vi "gui-camera-status-converter.vi"(1 "xenics-status-cluster":T1, 2 "andor-status-cluster":T4={"Newton Init"=FALSE, "Newton Cooling"=FALSE, "Newton Parameters "=FALSE, "iDus Init"=FALSE, "iDus Cooling"=FALSE, "iDus Parameters"=FALSE, "Clara Init"=FALSE, "Clara Cooling"=FALSE, "Clara Parameters"=FALSE, "Newton Cooler StatusCode"=enum."N/A (0)", "iDus Cooler StatusCode"=enum."N/A (0)", "Clara Cooler StatusCode"=enum."DRV_TEMPERATURE_NOT_REACHED"}) -> (0 "general-camera-status":T2)   [LabVIEW 2017]
uses:
  <userlib>/atmcd32d.llb/Error Code Enum typedef.ctl
panel:
  # "Init"
  # "Cooling"
  # "Parameters"
  # "Xeva"
  # "Init"
  # "Cooling"
  # "Parameters"
  # "Newton"
  # "iDus"
  # "Clara"
  # "Xeva"
  # "Init"
  # "Cooling"
  # "Parameters"
  # "Newton"
  # "iDus"
  # "Clara"
  # "Clara"
  # "iDus"
  # "Newton"
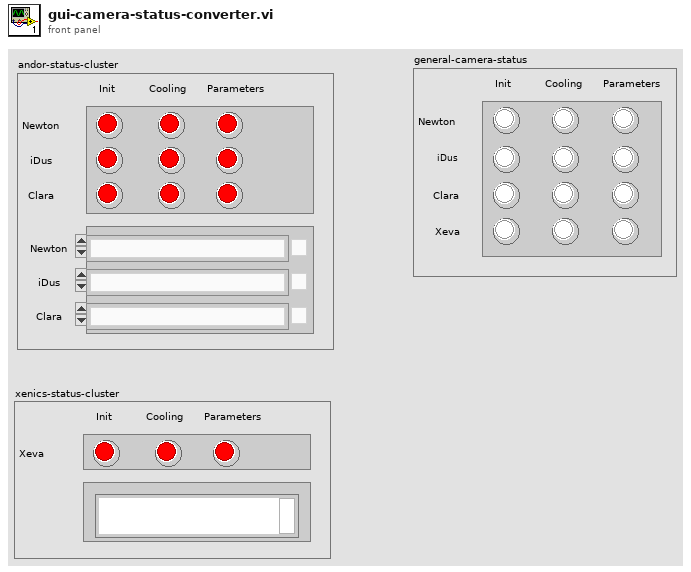
[diagram p1: front panel]
types:
  T1 = cluster{"Xeva-init":bool, "xeva-cooling":bool, "xeva-parameters":bool, "xeva-error":string}
  T2 = cluster{"Newton Init":bool, "Newton Cooling":bool, "Newton Parameters ":bool, "iDus Init":bool, "iDus Cooling":bool, "iDus Parameters":bool, "Clara Init":bool, "Clara Cooling":bool, "Clara Parameters":bool, "Xeva-init":bool, "xeva-cooling":bool, "xeva-parameters":bool}
  T3 = typedef "Error Code Enum typedef.ctl" = enum32{"N/A (0)", "DRV_ERROR_CODES", "DRV_SUCCESS", "DRV_VXDNOTINSTALLED", "DRV_ERROR_SCAN", "DRV_ERROR_CHECK_SUM", "DRV_ERROR_FILELOAD", "DRV_UNKNOWN_FUNC", "DRV_ERROR_VXD_INIT", "DRV_ERROR_ADDRESS", "DRV_ERROR_PAGELOCK", "DRV_ERROR_PAGEUNLOCK", "DRV_ERROR_BOARDTEST", "DRV_ERROR_ACK", "DRV_ERROR_UP_FIFO", "DRV_ERROR_PATTERN", "N/A (16)", "DRV_ACQUISITION_ERRORS", "DRV_ACQ_BUFFER", "DRV_ACQ_DOWNFIFO_FULL", "DRV_PROC_UNKONWN_INSTRUCTION", "DRV_ILLEGAL_OP_CODE", "DRV_KINETIC_TIME_NOT_MET", "DRV_ACCUM_TIME_NOT_MET", "DRV_NO_NEW_DATA", "N/A (25)", "DRV_SPOOLERROR", "N/A (27)", "N/A (28)", "N/A (29)", "N/A (30)", "N/A (31)", "N/A (32)", "DRV_TEMPERATURE_CODES", "DRV_TEMPERATURE_OFF", "DRV_TEMPERATURE_NOT_STABILIZED", "DRV_TEMPERATURE_STABILIZED", "DRV_TEMPERATURE_NOT_REACHED", "DRV_TEMPERATURE_OUT_RANGE", "DRV_TEMPERATURE_NOT_SUPPORTED", "DRV_TEMPERATURE_DRIFT", "N/A (41)", "N/A (42)", "N/A (43)", "N/A (44)", "N/A (45)", "N/A (46)", "N/A (47)", "N/A (48)", "DRV_GENERAL_ERRORS", "DRV_INVALID_AUX", "DRV_COF_NOTLOADED", "DRV_FPGAPROG", "DRV_FLEXERROR", "DRV_GPIBERROR", "N/A (55)", "N/A (56)", "N/A (57)", "N/A (58)", "N/A (59)", "N/A (60)", "N/A (61)", "N/A (62)", "N/A (63)", "DRV_DATATYPE", "DRV_DRIVER_ERRORS", "DRV_P1INVALID", "DRV_P2INVALID", "DRV_P3INVALID", "DRV_P4INVALID", "DRV_INIERROR", "DRV_COFERROR", "DRV_ACQUIRING", "DRV_IDLE", "DRV_TEMPCYCLE", "DRV_NOT_INITIALIZED", "DRV_P5INVALID", "DRV_P6INVALID", "DRV_INVALID_MODE", "DRV_INVALID_FILTER", "DRV_I2CERRORS", "DRV_I2CDEVNOTFOUND", "DRV_I2CTIMEOUT", "DRV_P7INVALID", "N/A (84)", "N/A (85)", "N/A (86)", "N/A (87)", "N/A (88)", "N/A (89)", "DRV_IOCERROR", "DRV_VRMVERSIONERROR"}
  T4 = cluster{"Newton Init":bool, "Newton Cooling":bool, "Newton Parameters ":bool, "iDus Init":bool, "iDus Cooling":bool, "iDus Parameters":bool, "Clara Init":bool, "Clara Cooling":bool, "Clara Parameters":bool, "Newton Cooler StatusCode":T3, "iDus Cooler StatusCode":T3, "Clara Cooler StatusCode":T3}
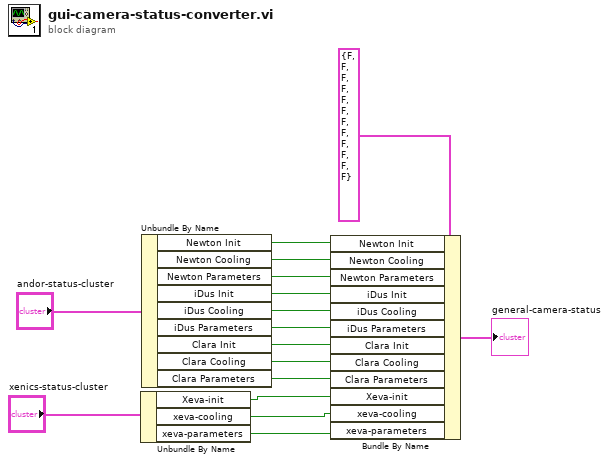
[diagram p0: block diagram]
diagram:
  n1 = Unbundle By Name("xenics-status-cluster") -> ("Xeva-init"=w11:bool, "xeva-cooling"=w10:bool, "xeva-parameters"=w9:bool)
  n2 = Unbundle By Name("andor-status-cluster") -> ("Newton Init"=w16:bool, "Newton Cooling"=w4:bool, "Newton Parameters"=w5:bool, "iDus Init"=w6:bool, "iDus Cooling"=w7:bool, "iDus Parameters"=w8:bool, "Clara Init"=w15:bool, "Clara Cooling"=w14:bool, "Clara Parameters"=w13:bool)
  n3 = Bundle By Name(cluster=T2 {"Newton Init"=FALSE, "Newton Cooling"=FALSE, "Newton Parameters "=FALSE, "iDus Init"=FALSE, "iDus Cooling"=FALSE, "iDus Parameters"=FALSE, "Clara Init"=FALSE, "Clara Cooling"=FALSE, "Clara Parameters"=FALSE, "Xeva-init"=FALSE, "xeva-cooling"=FALSE, "xeva-parameters"=FALSE} ("general-camera-status"), "Newton Init"=w16, "Newton Cooling"=w4, "Newton Parameters"=w5, "iDus Init"=w6, "iDus Cooling"=w7, "iDus Parameters"=w8, "Clara Init"=w15, "Clara Cooling"=w14, "Clara Parameters"=w13, "Xeva-init"=w11, "xeva-cooling"=w10, "xeva-parameters"=w9) -> (→"general-camera-status":T2)
